vi "WPI_InterruptCache.vi"(8 "error in (no error)":errorcluster, 9 "InterruptIndexToRelease":T1, 11 "InterruptCacheOp":T2) -> (0 "error out":errorcluster, 2 "InterruptIndexAllocated":T1, 3 "Allocated":bool)   [LabVIEW 2017]
doc: "This software is licensed. Open the labview\\readme\\WPI Robotics Library Open Source License.txt file for more information."
uses:
  <vilib>/Rock Robotics/WPI/Interrupt/WPI_InterruptCacheOp.ctl
  <vilib>/Rock Robotics/SystemInterfaces/Interrupt/FPGA_InterruptIndex.ctl
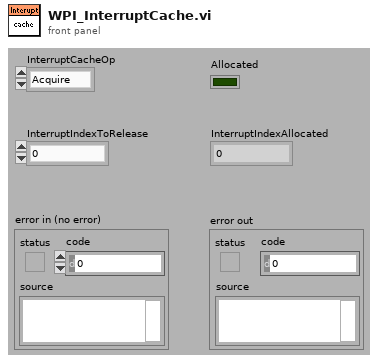
[diagram p1: front panel]
types:
  T1 = typedef "FPGA_InterruptIndex.ctl" = enum8{"0", "1", "2", "3", "4", "5", "6", "7", "Invalid"}
  T2 = typedef "WPI_InterruptCacheOp.ctl" = enum16{"Acquire", "Release"}
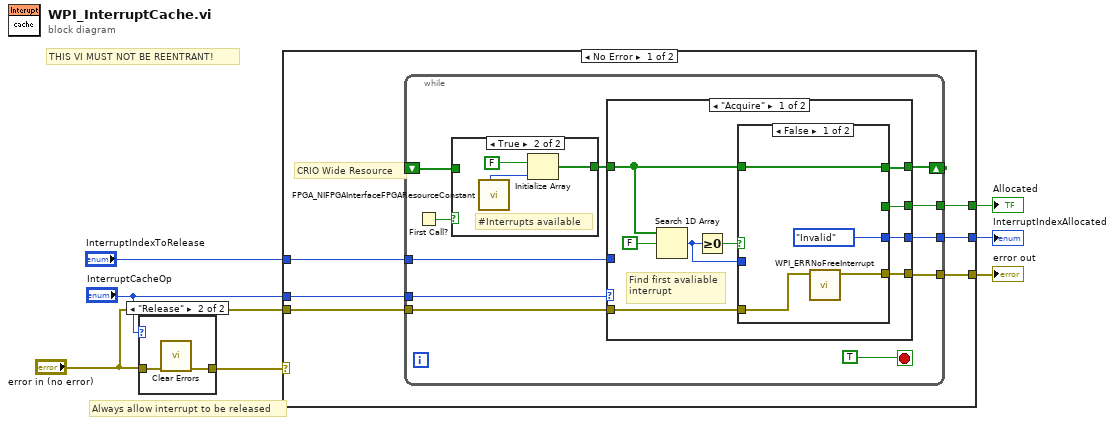
[diagram p0: block diagram]
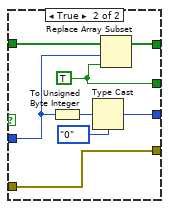
[diagram p3: hidden frame]
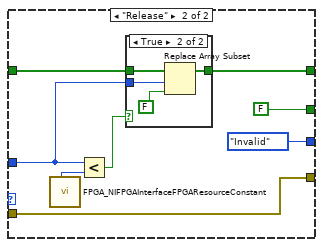
[diagram p4: hidden frame]
diagram:
  # "THIS VI MUST NOT BE REENTRANT!"
  # "Always allow interrupt to be released"
  n1 = case shown="\"Release\"" "InterruptCacheOp" {
    tunnel: "error in (no error)" -> [w8 w10]
    tunnel: [w8 w9] -> w5
    frame "Acquire", Default {
    }
    frame "Release" {
      n2 = call <vilib>:"Clear Errors.vi"("error in (no error)"=w10) -> ("error out"=w9:errorcluster)  [unwired: 1 in, 5 out]
    }
  }
  n3 = case shown="No Error" w5 {
    selector: w5 -> [_ w66]
    tunnel: "InterruptCacheOp" -> [w16 _]
    tunnel: [w15 w66] -> w1
    tunnel: [w14 _] -> w7
    tunnel: "InterruptIndexToRelease" -> [w12 _]
    tunnel: [w13 _] -> w3
    tunnel: "error in (no error)" -> [w11 _]
    frame No Error {
      # "CRIO Wide Resource"
      n4 = while {
        shift-right: [w24] -> _
        shift-left: _ -> [w26]
        tunnel: w16 -> [w25]
        tunnel: w12 -> [w20]
        tunnel: [w23] -> w15
        tunnel: [w22] -> w14
        tunnel: [w19] -> w13
        tunnel: w11 -> [w17]
        stop <- TRUE stop-if-true
        n5 = First Call?() -> (First Call?: T/F=w27:bool)
        n6 = case shown="True" w27 {
          tunnel: w26 -> [w62 _]
          tunnel: [w62 w64] -> w21
          frame False {
          }
          frame True {
            # "#Interrupts available"
            n7 = call <vilib>:"FPGA_NIFPGAInterfaceFPGAResourceConstant.vi"() -> ("NumberOfInterrupts"=w63:u32)  [unwired: 11 out]
            n8 = Initialize Array(FALSE, w63) -> (w64:bool[])
          }
        }
        n9 = case shown="\"Acquire\"" w25 {
          tunnel: w21 -> [w32 w56]
          tunnel: [w36 w55] -> w24
          tunnel: w20 -> [_ w53]
          tunnel: [w35 w54] -> w23
          tunnel: [w34 FALSE ("new element/subarray")] -> w22
          tunnel: [w33 FPGA_InterruptIndex."Invalid" ("InterruptIndexToRelease")] -> w19
          tunnel: w17 -> [w28 w54]
          frame "Acquire" {
            # "Find first avaliable\ninterrupt"
            n10 = Search 1D Array(1D array=w32, element=FALSE) -> (index of element=w29:i32)  [unwired: 1 out]
            n11 = Greater Or Equal To 0?(x=w29) -> (x >= 0?=w30:bool)
            n12 = case shown="False" w30 {
              tunnel: w32 -> [w40 w47]
              tunnel: [w40 w46] -> w36
              tunnel: w29 -> [_ w42]
              tunnel: [w37 w43] -> w35
              tunnel: [_ w48] -> w34
              tunnel: [FPGA_InterruptIndex."Invalid" ("InterruptIndexToRelease") w45] -> w33
              tunnel: w28 -> [w38 w43]
              frame False {
                n13 = call <vilib>:"WPI_ERRNoFreeInterrupt.vi"("error in (no error)"=w38) -> ("InteruptAllocation"=w37:errorcluster)  [unwired: 10 out]
              }
              frame True {
                w48 = TRUE ("new element/subarray")
                n14 = To Unsigned Byte Integer(number=w42) -> (unsigned 8bit integer=w44:u8)
                n15 = Type Cast(type=FPGA_InterruptIndex."0" ("InterruptIndexToRelease"), x=w44) -> (*(type *) &x=w45:T1)
                n16 = Replace Array Subset(array=w47, new element=w48, index=w42) -> (w46:bool[])
              }
            }
          }
          frame "Release" {
            n17 = call <vilib>:"FPGA_NIFPGAInterfaceFPGAResourceConstant.vi"() -> ("NumberOfInterrupts"=w52:u32)  [unwired: 11 out]
            n18 = Less?(x=w53, y=w52) -> (x < y?=w51:bool)
            n19 = case shown="True" w51 {
              tunnel: w56 -> [w57 w61]
              tunnel: [w57 w60] -> w55
              tunnel: w53 -> [_ w59]
              frame False {
              }
              frame True {
                n20 = Replace Array Subset(array=w61, new element=FALSE ("new element/subarray"), index=w59) -> (w60:bool[])
              }
            }
          }
        }
      }
    }
    frame Error {
    }
  }
  "Allocated" <- w7
  "error out" <- w1
  "InterruptIndexAllocated" <- w3
